vi "Optionen initialisieren.vi"(8 "error in (no error)":errorcluster caption="Fehler (Eingang, kein Fehler)", 11 "Cluster (Eingang)":refnum<vi>) -> (0 "Fehler (Ausgang)":errorcluster, 3 "Wartungsintervall:":sgl)   [LabVIEW 2020, in "System Einstellungen V2.lvlib"]
uses:
  System Einstellungen V2.lvlib
  Aktion FGV SystemEinstellungenV2.ctl
  Aktioen FGV System.ctl
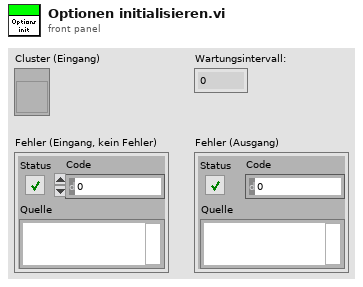
[diagram p1: front panel]
types:
  T1 = typedef "System Einstellungen V2.lvlib/Aktioen FGV System.ctl" = enum16{"lesen", "laden", "speichern", "Optionen schreiben", "Zeitstempel", "Reset BMP", "Reset SQP", "Wartung", "Werkseinstellung"}
  T2 = typedef "System Einstellungen V2.lvlib/Aktion FGV SystemEinstellungenV2.ctl" = enum16{"lesen", "Analysatoren schreiben", "Analysator ändern", "Analysatoren löschen", "laden", "speichern", "Untertitel", "Analysatoren", "Neue Analysatoren", "Gasteiler schreiben", "Gasteiler ändern", "Gasteiler löschen", "Gasteiler", "Gasteiler exportieren", "Gasteiler importieren"}
  T3 = typedef "System Einstellungen V2.lvlib/Optionen.ctl" = cluster{"Störmeldep.":bool, "Betriebszustände":bool, "AK in ppm":bool, "log Cal-Gas":bool, "log 0-Gas":bool, "Durchflusssensor 0-5V":bool, "PNS?":bool, "Mit N2 spülen":bool, "TRE08":bool, "Amium 10-Fach":bool, "Verticale Scrollbar aktiv":bool, "Loggingtakt":bool, "AK Rezeptwechsel gleich wie MKS":bool, "NG ECO":bool}
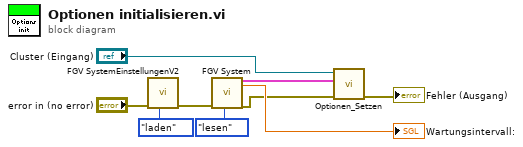
[diagram p0: block diagram]
diagram:
  n1 = call "FGV SystemEinstellungenV2.vi"("Aktion"=Aktion_FGV_SystemEinstellungenV2."laden", "error in (no error)"="error in (no error)") -> ("error out"=w7:errorcluster)  [unwired: 4 in, 5 out]
  n2 = call "FGV System.vi"("error in (no error)"=w7, "Aktionen"=Aktioen_FGV_System."lesen") -> ("Optionen"=w4:T3, "Wartungsintervall:"=→"Wartungsintervall:":sgl, "error out"=w8:errorcluster)  [unwired: 11 in, 4 out]
  n3 = call "Optionen_Setzen.vi"("error in (no error)"=w8, "Optionen (Eingang)"=w4, "Optionen Anzeige (Eingang)"="Cluster (Eingang)") -> ("error out"=→"Fehler (Ausgang)":errorcluster)  [unwired: 8 in]
